vi "measure_z_voltage.vi"(8 "error in":errorcluster, 11 "Coarse Approach in":refnum<class "Coarse Approach.lvclass">) -> (0 "error out":errorcluster, 2 "Z Voltage out":i16(slide) scale=32767.0..-32768.0, 3 "Coarse Approach out":refnum<class "Coarse Approach.lvclass">)   [LabVIEW 2020, in "Coarse Approach.lvclass"]
uses:
  Coarse Approach.lvclass
  Coarse Approach.lvclass/Coarse Approach.ctl
  PZT/PZT.lvclass
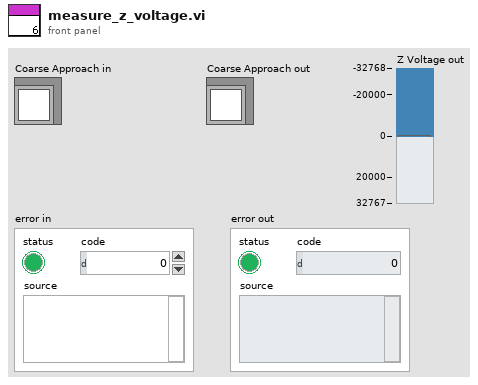
[diagram p1: front panel]
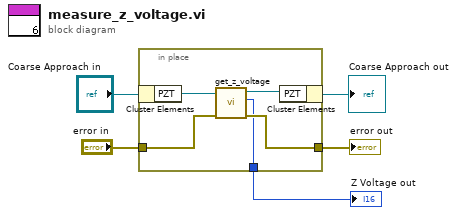
[diagram p0: block diagram]
diagram:
  n1 = in-place {
    in-place-border: "error in" -> [w8]
    in-place-border: [w7] -> w2
    in-place-border: [w6] -> w1
    n2 = in-place-cluster #1("Coarse Approach in") -> ("PZT"=w10:refnum<class "PZT.lvclass">)
    n3 = call "get_z_voltage.vi"("error in"=w8, "PZT in"=w10) -> ("error out"=w7:errorcluster, "Z Voltage out"=w6:i16, "PZT out"=w9:refnum<class "PZT.lvclass">)  [unwired: 7 in]
    n4 = in-place-cluster #1("PZT"=w9) -> (→"Coarse Approach out":refnum<class "Coarse Approach.lvclass">)
  }
  "error out" <- w2
  "Z Voltage out" <- w1
